vi "Insert VI.vi"(8 "error in (no error)":errorcluster, 10 "VIRef":refnum<vi>, 11 "TabControl in":refnum<vi>) -> (0 "error out":errorcluster, 3 "TabControl out":refnum<vi>)   [LabVIEW 2020, in "MDI ViewManager.lvlib"]
uses:
  MDI ViewManager.lvlib
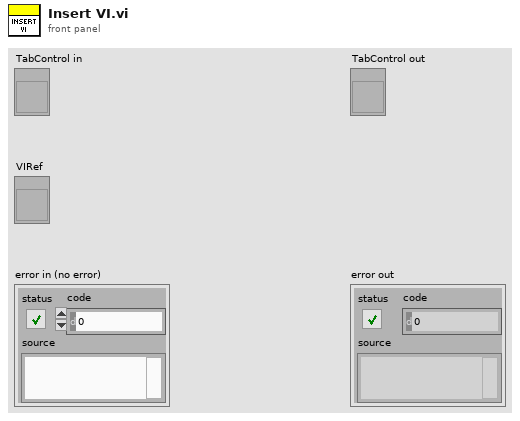
[diagram p1: front panel]
types:
  T1 = enum32{"Invalid", "Standard", "Closed", "Hidden", "Minimized", "Maximized"}
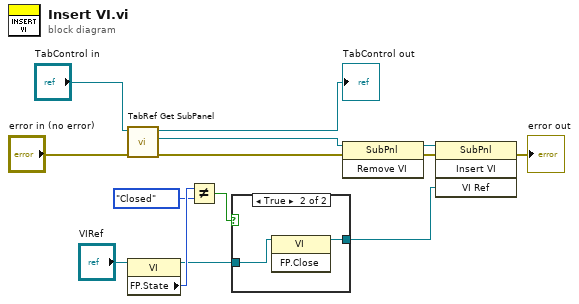
[diagram p0: block diagram]
diagram:
  n1 = call "TabRef Get SubPanel.vi"("error in (no error)"="error in (no error)", "TabControl in"="TabControl in") -> ("error out"=w2:errorcluster, "Sub Panel"=w13:refnum<vi>, "TabControl out"=→"TabControl out":refnum<vi>)  [unwired: 7 in]
  n2 = property class="VI"(reference="VIRef") -> (reference out=w9:refnum<vi>, "FP.State"=w12:T1)  [unwired: 1 in, 1 out]
  n3 = Not Equal?(x=w12, y=T1."Closed") -> (x != y?=w10:bool)
  n4 = case shown="True" w10 {
    tunnel: w9 -> [w15 w17]
    tunnel: [w15 w16] -> w8
    frame False {
    }
    frame True {
      n5 = invoke class="VI" method="FP.Close"(reference=w17) -> (reference out=w16:refnum<vi>)  [unwired: 2 in, 2 out]
    }
  }
  n6 = invoke class="SubPnl" method="Remove VI"(reference=w13, error in=w2) -> (reference out=w7:refnum<vi>, error out=w6:errorcluster)  [unwired: 1 in, 1 out]
  n7 = invoke class="SubPnl" method="Insert VI"(reference=w7, error in=w6, "VI Ref"=w8) -> (error out=→"error out":errorcluster)  [unwired: 1 in, 3 out]
